vi "Troca.vi"(10 "first call":bool, 11 "InfoMissao":T1 {"Agentes Disponíveis" format="%#_13g"}) -> (3 "Vetor de Agentes":i32[](array[numeric]))   [LabVIEW 2018]
uses:
  InfoMissao.ctl
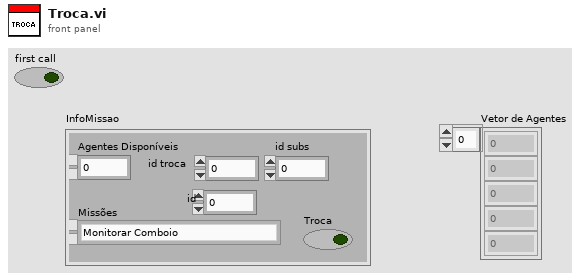
[diagram p1: front panel]
types:
  T1 = typedef "InfoMissao.ctl" = cluster{"Troca ":bool, "Missões ":enum16{"Monitorar Comboio", "Realizar Segurança de Retaguarda", "Vigiar Área", "Reconhecimento de Área"}, "Agentes Disponíveis":dbl, "id troca ":dbl, "id subs":dbl, "id ":dbl}
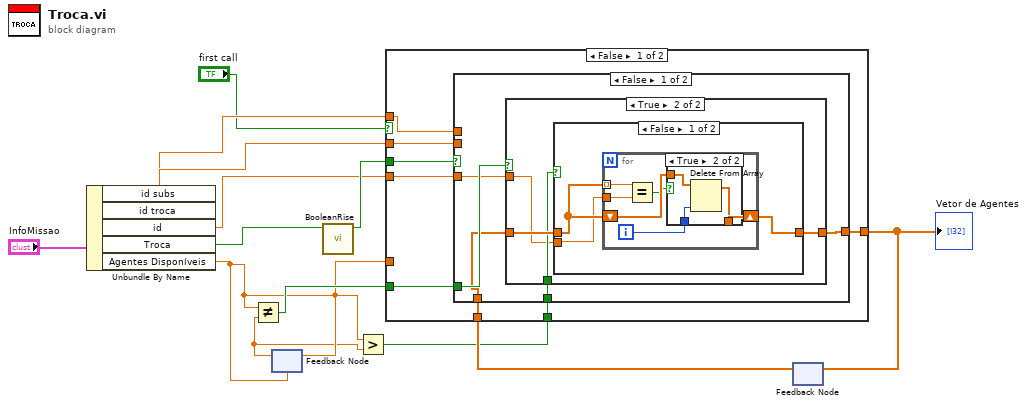
[diagram p0: block diagram]
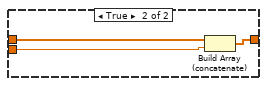
[diagram p4: hidden frame]
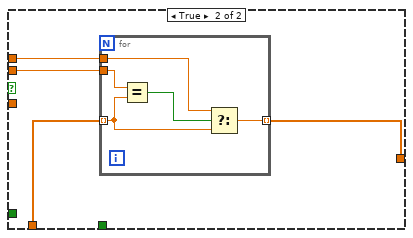
[diagram p5: hidden frame]
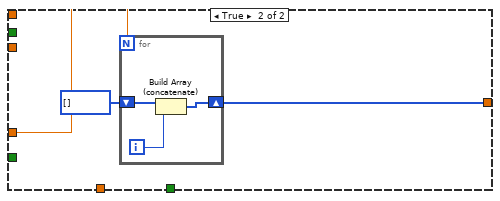
[diagram p6: hidden frame]
diagram:
  n1 = Unbundle By Name("InfoMissao") -> ("id subs"=w7:dbl, "id troca"=w8:dbl, "id"=w4:dbl, "Troca"=w12:bool, "Agentes Disponíveis"=w3:dbl)
  n2 = feedback-in #1(w3) -> ()
  n3 = feedback #1(w3) -> (w2:dbl)
  n4 = Not Equal?(x=w3, y=w2) -> (x != y?=w5:bool)
  n5 = call "BooleanRise.vi"("Test Mode On"=w12) -> ("Boolean"=w11:bool)  [unwired: 10 in]
  n6 = Greater?(x=w3, y=w2) -> (0:w1:bool)
  n7 = feedback #2() -> (w9:dbl[])  [unwired: 1 in]
  n8 = case shown="False" "first call" {
    tunnel: w3 -> [_ w59]
    tunnel: [w20 w57] -> w10
    tunnel: w11 -> [w21 _]
    tunnel: w9 -> [w19 _]
    tunnel: w8 -> [w18 _]
    tunnel: w7 -> [w17 _]
    tunnel: w5 -> [w16 _]
    tunnel: w4 -> [w15 _]
    tunnel: w1 -> [w14 _]
    frame False {
      n9 = case shown="False" w21 {
        tunnel: [w25 w49] -> w20
        tunnel: w19 -> [w24 w51]
        tunnel: w18 -> [_ w50]
        tunnel: w17 -> [_ w48]
        tunnel: w16 -> [w26 _]
        tunnel: w15 -> [w23 _]
        tunnel: w14 -> [w22 _]
        frame False {
          n10 = case shown="True" w26 {
            tunnel: [w27 w28] -> w25
            tunnel: w24 -> [w27 w31]
            tunnel: w23 -> [_ w29]
            tunnel: w22 -> [_ w30]
            frame False {
            }
            frame True {
              n11 = case shown="False" w30 {
                tunnel: w31 -> [w34 w47]
                tunnel: w29 -> [w32 w46]
                tunnel: [w33 w45] -> w28
                frame False {
                  n12 = for {
                    tunnel: w34 -> [w40] mode=indexing
                    tunnel: w32 -> [w39]
                    shift-right: [w36] -> w33
                    shift-left: w34 -> [w38]
                    i -> [w37]
                    n13 = Equal?(x=w40, y=w39) -> (x = y?=w35:bool)
                    n14 = case shown="True" w35 {
                      tunnel: w38 -> [w41 w44]
                      tunnel: w37 -> [_ w43]
                      tunnel: [w41 w42] -> w36
                      frame False {
                      }
                      frame True {
                        n15 = Delete From Array(array=w44, index=w43) -> (array with subset deleted=w42:dbl[])  [unwired: 1 in, 1 out]
                      }
                    }
                  }
                }
                frame True {
                  n16 = Build Array (concatenate)(w47, w46) -> (w45:dbl[])
                }
              }
            }
          }
        }
        frame True {
          n17 = for {
            tunnel: w51 -> [w55] mode=indexing
            tunnel: w50 -> [w54]
            tunnel: [w53] -> w49 mode=indexing
            tunnel: w48 -> [w52]
            n18 = Equal?(x=w54, y=w55) -> (x = y?=w56:bool)
            n19 = Select(t=w52, s=w56, f=w55) -> (s? t:f=w53:dbl)
          }
        }
      }
    }
    frame True {
      n20 = for {
        N: w59 -> [_]
        shift-right: [w61] -> w57
        shift-left: i32[] [] -> [w60]
        i -> [w62]
        n21 = Build Array (concatenate)(w60, w62) -> (w61:i32[])
      }
    }
  }
  "Vetor de Agentes" <- w10
  n22 = feedback-in #2(w10) -> ()
